vi "Connect List.vi"(8 "error in (no error)":errorcluster, 10 "Params":variant, 11 "PIPXI40 Switching in":refnum<class "PIPX40 Relay.lvclass">) -> (0 "error out":errorcluster, 3 "PIPXI40 Switching out":refnum<class "PIPX40 Relay.lvclass">)   [LabVIEW 2020, in "Pickering.lvlib" / "PIPX40 Relay.lvclass"]
uses:
  PIPX40 Relay.lvclass
  D:/WSGitHub/RTFWK/Realization/PIPX40 Base/PIPX40 Base.lvclass
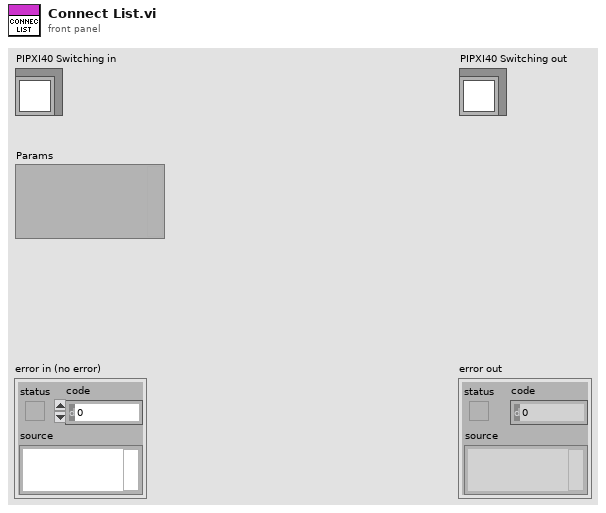
[diagram p1: front panel]
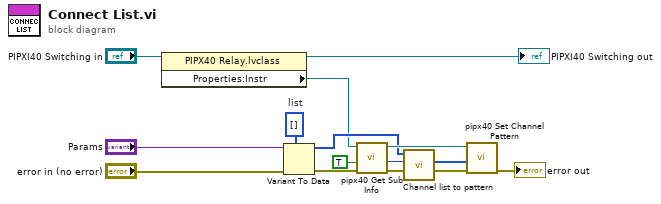
[diagram p0: block diagram]
diagram:
  w7 = i32[] []  # list
  n1 = property class="PIPX40 Relay.lvclass"(reference="PIPXI40 Switching in") -> (reference out=→"PIPXI40 Switching out":refnum<class "PIPX40 Relay.lvclass">, "Properties:Instr"=w2:refnum<visa-resource-name>)  [unwired: 1 in, 1 out]
  n2 = Variant To Data(error in="error in (no error)", type=w7, Variant="Params") -> (data=w5:i32[], error out=w11:errorcluster)
  n3 = call <instrlib>:"pipx40 Get Sub Info.vi"("error in (no error)"=w11, "is output"=TRUE, "instrument handle"=w2) -> ("error out"=w10:errorcluster, "columns"=w9:u32, "instrument handle out"=w8:refnum<visa-resource-name>)  [unwired: 4 in, 2 out]
  n4 = call "Channel list to pattern.vi"("Outputs"=w9, "List"=w5) -> ("Pattern"=w4:u32[])  [unwired: 9 in]
  n5 = call <instrlib>:"pipx40 Set Channel Pattern.vi"("error in (no error)"=w10, "pattern"=w4, "instrument handle"=w8) -> ("error out"=→"error out":errorcluster)  [unwired: 7 in, 1 out]
